vi "Main.vi"() -> ()   [LabVIEW 2014, in "GenNet-Client.lvlib"]
doc: "The GenNet-Client module is instantiated from a DQMH Generic Networking Module\nin order to forward messages via TCP/IP.\n\nThe GenNet-Client module forwards all requests to another DQMH Generic Networking \nModule running in another application and/or another PC accessible via TCP/IP.\n\n<b>Note:</b> This VI was modified by the <b>Validate DQMH Module</b> tool to upgrade it to the DQMH 5.0 approach to destroying cloneable module event references.\n\n<b>Note:</b> This VI was modified by the <b>Validate DQMH Module</b> tool to have the module name be passed as the Additional Information parameter with an Error Reported broadcast.\n\n<b>Note:</b> This VI was modified by the <b>Validate DQMH Module</b> tool to call the Release Message Queue VI in the top-level Error case.\n\n<b>Note:</b> This VI was modified by the <b>Validate DQMH Module</b> tool to call the Release Message Queue VI in the top-level Error case."
uses:
  GenNet-Client.lvlib
  <vilib>/Delacor/Delacor QMH/Libraries/Cloneable Module Admin_class/Delacor_lib_QMH_Cloneable Module Admin.lvclass
  DQMH-GenNet Message Queue.lvclass
  hse-dqmh/Controls/System Message Argument--cluster.ctl
  hse-dqmh/Controls/System Message Source.ctl
  Module Data--cluster.ctl
  Stop Argument--cluster.ctl
  <vilib>/Delacor/Delacor QMH/Libraries/Message Queue_class/Delacor_lib_QMH_Message Queue.lvclass/Delacor_lib_QMH_Message Queue.ctl
  <vilib>/Delacor/Delacor QMH/Libraries/Cloneable Module Admin_class/Delacor_lib_QMH_Cloneable Module Admin.lvclass/Delacor_lib_QMH_Cloneable Module Admin.ctl
  <vilib>/Delacor/Delacor QMH/Libraries/Module Admin_class/Delacor_lib_QMH_Module Admin.lvclass/Delacor_lib_QMH_Module Admin.ctl
  Connect Argument--cluster.ctl
  Connect (Reply Payload)--cluster.ctl
  Send via Network Argument--cluster.ctl
  Listen for Network Broadcasts Argument--cluster.ctl
  <vilib>/Utility/miscctls.llb/LVPointTypeDef.ctl
  <vilib>/Delacor/Delacor QMH/Libraries/Message Queue_class/Delacor_lib_QMH_Enqueue Message (Single).vi
  <vilib>/Delacor/Delacor QMH/Libraries/Cloneable Module Admin_class/Delacor_lib_QMH_Get Module ID.vi
  <vilib>/Delacor/Delacor QMH/Libraries/Module Admin_class/Delacor_lib_QMH_Get External Launch.vi
  <vilib>/Utility/tcp.llb/UDP Multicast Read-Only Open.vi
  <vilib>/Utility/error.llb/Error Cluster From Error Code.vi
  <vilib>/ErrorRing/Error Ring.xnode
  <vilib>/Delacor/Delacor QMH/Libraries/Message Queue_class/Delacor_lib_QMH_Message Queue.lvclass
  hse-gennet.lvlib
  hse-dqmh/hse-dqmh.lvlib
panel:
  in  "Call Chain":string[](array[string])
  in  "Caller SystemMsg":refnum<user-event>
  in  "Caller MsgQ":refnum<class "DQMH-GenNet Message Queue.lvclass">
  out "error out":errorcluster
  in  "Module Admin":refnum<class "Delacor_lib_QMH_Cloneable Module Admin.lvclass">
  # "The GenNet-Client module is instantiated from a DQMH Generic Networking Module\nin order to forward messages via TCP/IP.\n\nThe GenNet-Client module forwards all requests to another DQMH Generic Networking \nModule running in another application and/or another PC accessible via TCP/IP."
  # "hse-lib.lvlib:System Message Argument--cluster.ctlCaveat:\nThe Caller's message queue, which should be private to the caller only, is avail-\nable to the GenNet-Server module so that it can write messages directly. As the GenNet-Server\nmodule cannot be accessed from other code, and as messages that arrive via\nnetwork are to be considered local, this excemption to the rule is tolerable."
  # "Please get in touch with us at office@hampel-soft.com or visit our website www.hampel-soft.com"
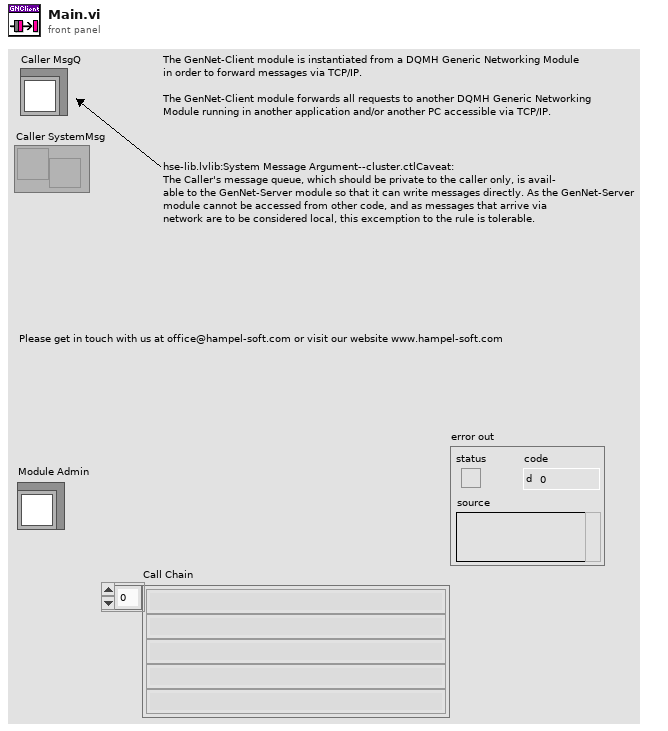
[diagram p1: front panel]
types:
  T1 = typedef "GenNet-Client.lvlib/Request Events--cluster.ctl" = cluster{"Stop Module":refnum<user-event>, "Show Panel":refnum<user-event>, "Hide Panel":refnum<user-event>, "Show Diagram":refnum<user-event>, "Get Module Execution Status":refnum<user-event>, "Send via Network":refnum<user-event>, "Connect":refnum<user-event>, "Listen for Network Broadcasts":refnum<user-event>}
  T2 = typedef "GenNet-Client.lvlib/Module Data--cluster.ctl" = cluster{"Status":string, "IP":string, "Port":u16, "Timeout":i32, "ConnID":refnum<k5>, "UDP ConnID":refnum<k16>, "TCP error":errorcluster}
  T3 = enum32{"invalid lock state", "Not Locked", "Locked (No Password)", "Password-protected"}
  T4 = typedef "GenNet-Client.lvlib/Stop Argument--cluster.ctl" = cluster{"Origin":string, "Module ID":i32, "Exit via Stop Module Req?":bool, "Wait for Module to stop?":bool}
  T5 = typedef "GenNet-Client.lvlib/Connect Argument--cluster.ctl" = cluster{"Module ID":i32, "Wait Notifier":refnum<notifier>}
  T6 = typedef "GenNet-Client.lvlib/Send via Network Argument--cluster.ctl" = cluster{"Module ID":i32, "Message Data":variant}
  T7 = typedef "hse-dqmh.lvlib/System Message Argument--cluster.ctl" = cluster{"Identifier":string, "Payload":variant, "Source Type":T8, "Source Name":string}
  T8 = typedef "hse-dqmh.lvlib/System Message Source.ctl" = enum16{"module", "application", "network"}
  T9 = typedef "GenNet-Client.lvlib/Listen for Network Broadcasts Argument--cluster.ctl" = cluster{"Module ID":i32, "Multicast Address":string, "Port":u16, "Local IP Address":string, "Max Rx Byte Size":i32}
  T10 = typedef "LVPointTypeDef.ctl" = cluster{"Horizontal":i16, "Vertical":i16}
  T11 = enum32{"Invalid", "Standard", "Closed", "Hidden", "Minimized", "Maximized"}
  T12 = typedef "GenNet-Client.lvlib/Connect (Reply Payload)--cluster.ctl" = cluster{"error":errorcluster}
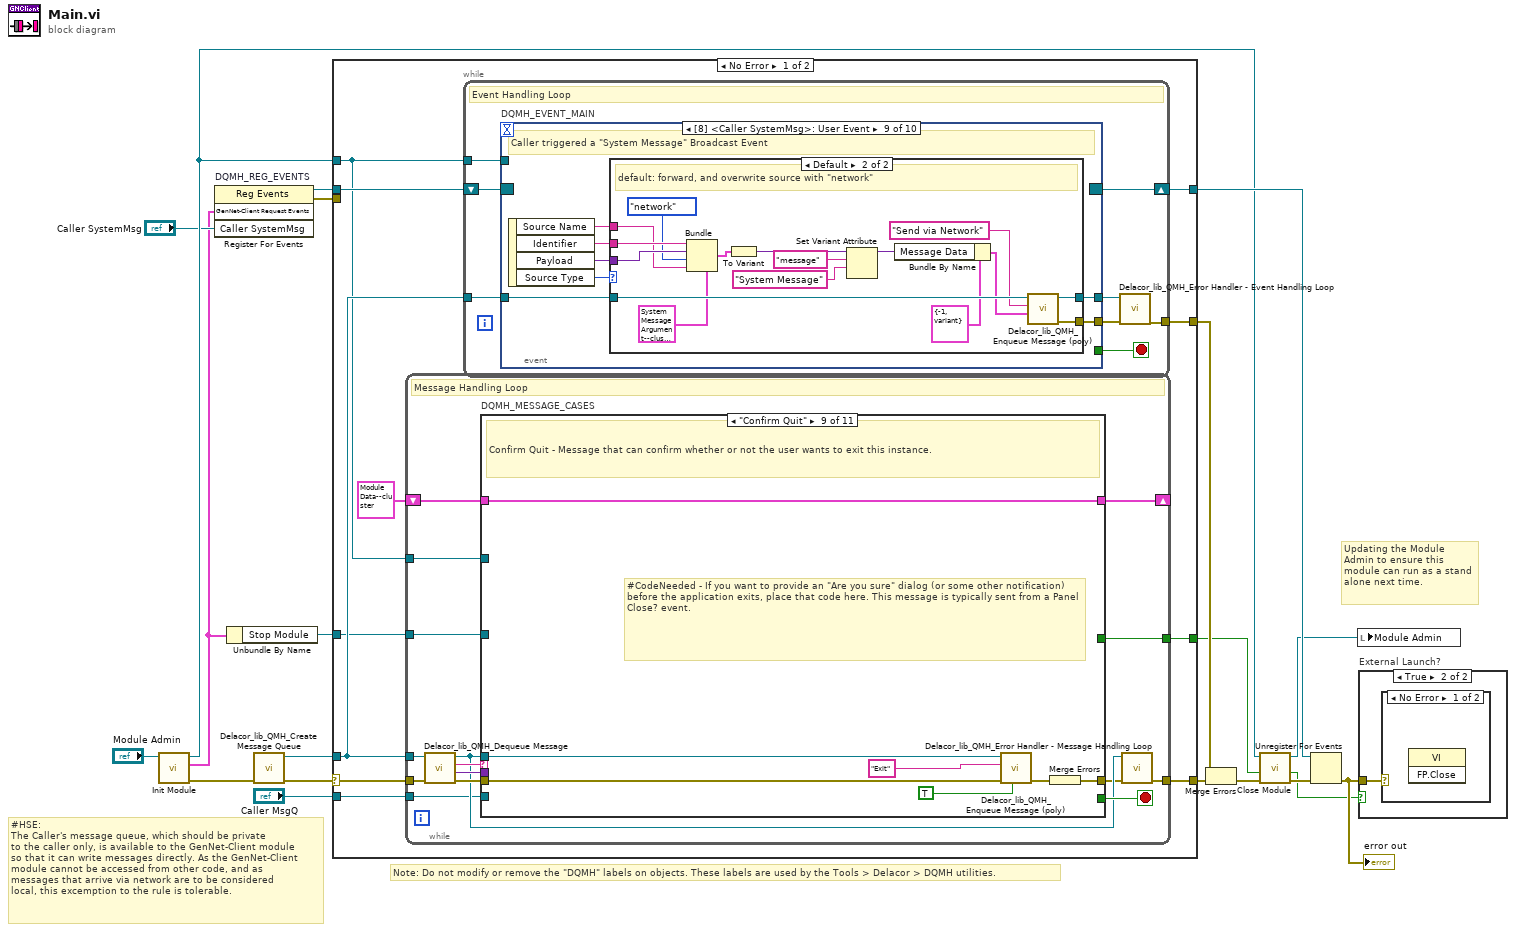
[diagram p0: block diagram]
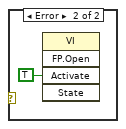
[diagram p3: hidden frame]
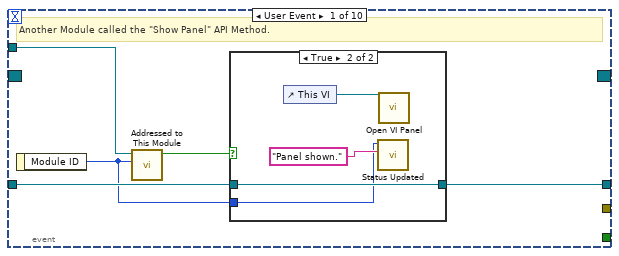
[diagram p4: hidden frame]
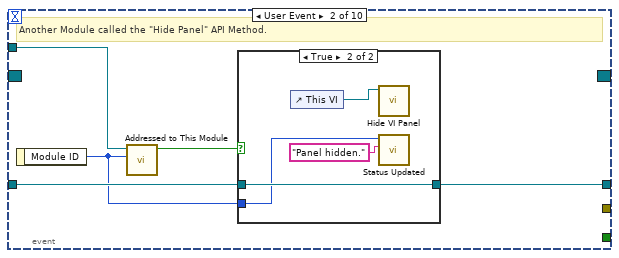
[diagram p6: hidden frame]
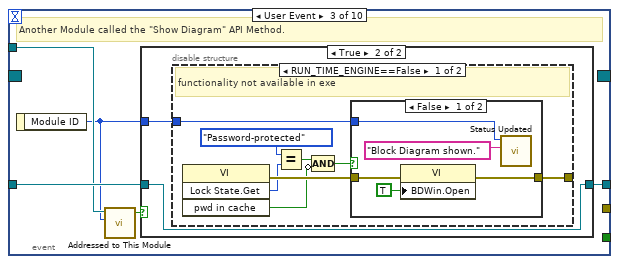
[diagram p8: hidden frame]
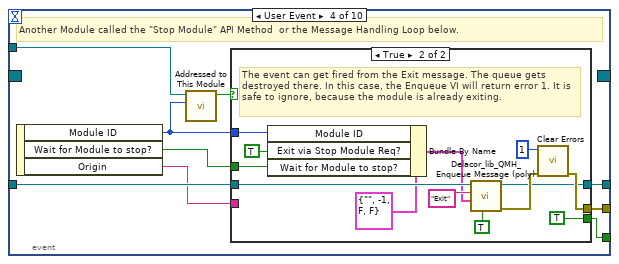
[diagram p12: hidden frame]
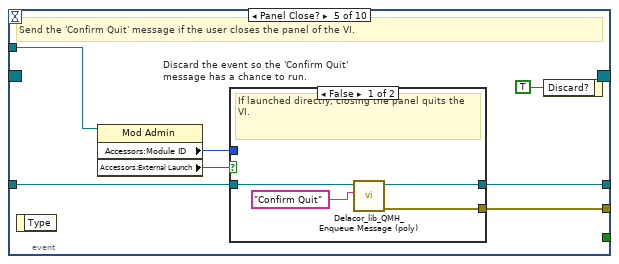
[diagram p14: hidden frame]
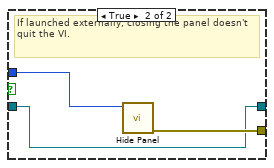
[diagram p15: hidden frame]
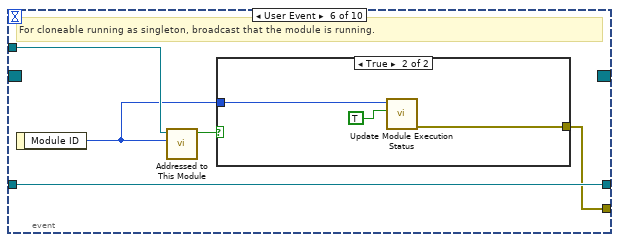
[diagram p16: hidden frame]
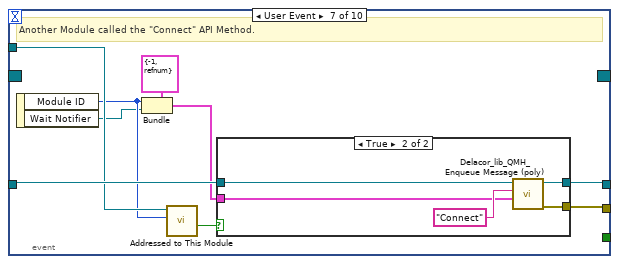
[diagram p18: hidden frame]
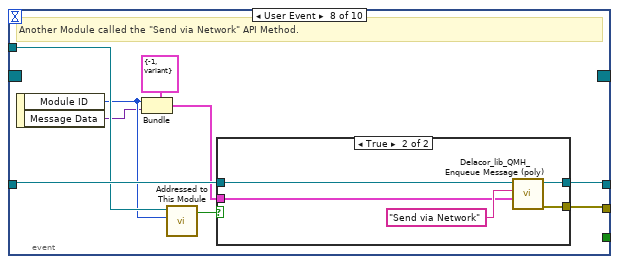
[diagram p20: hidden frame]
diagram:
  # "#HSE: \nThe Caller's message queue, which should be private \nto the caller only, is available to the GenNet-Client module \nso that it can write messages directly. As the GenNet-Client\nmodule cannot be accessed from other code, and as \nmessages that arrive via network are to be considered \nlocal, this excemption to the rule is tolerable."
  # "Note: Do not modify or remove the \"DQMH\" labels on objects. These labels are used by the Tools > Delacor > DQMH utilities."
  # "Updating the Module Admin to ensure this module can run as a stand alone next time."
  n1 = call "Init Module.vi"("Cloneable Module Admin in"="Module Admin") -> ("error out"=w17:errorcluster, "GenNet-Client Request Events"=w2:T1, "Cloneable Module Admin out"=w11:refnum<class "Delacor_lib_QMH_Cloneable Module Admin.lvclass">)  [unwired: 8 in]
  n2 = register-events "DQMH_REG_EVENTS"(w2, "Caller SystemMsg") -> (reference out=w15:refnum<event-registration>, error out=w4:errorcluster)  [unwired: 2 in]
  n3 = Unbundle By Name(w2) -> ("Stop Module"=w1:refnum<user-event>)
  n4 = call <vilib>:"Delacor_lib_QMH_Create Message Queue.vi"("error in (no error)"=w17) -> ("error out"=w6:errorcluster, "Message Queue"=w14:refnum<class "Delacor_lib_QMH_Message Queue.lvclass">)  [unwired: 9 in]
  n5 = case shown="No Error" w6 {
    selector: w6 -> [w25 w377]
    tunnel: [w31 w377] -> w18
    tunnel: [w30 w378] -> w16
    tunnel: w15 -> [w28 w378]
    tunnel: w14 -> [w27 w370]
    tunnel: [w26 _] -> w19
    tunnel: w11 -> [w24 w373]
    tunnel: [w23 _] -> w9
    tunnel: "Caller MsgQ" -> [w22 w369]
    tunnel: w4 -> [_ _]
    tunnel: w1 -> [w21 _]
    frame No Error {
      n6 = while {
        tunnel: w27 -> [w207]
        shift-right: [w213] -> _
        shift-left: T2 {"Status"="", "IP"="", "Port"=0, "Timeout"=0, "ConnID"=refnum, "UDP ConnID"=refnum, "TCP error"={"status"=FALSE, "code"=0, "source"=""}} ("Data Cluster") -> [w200]
        tunnel: w25 -> [w211]
        tunnel: [w205] -> w31
        tunnel: w24 -> [w204]
        tunnel: [w203] -> w23
        tunnel: w22 -> [w202]
        tunnel: w21 -> [w199]
        stop <- w212 stop-if-true
        # "Message Handling Loop"
        n7 = call-dynamic "Delacor_lib_QMH_Dequeue Message.vi"("error in (no error)"=w211, "Message Queue in"=w207) -> ("error out"=w210:errorcluster, "Message Data"=w208:variant, "Message"=w209:string, "Message Queue out"=w206:refnum<class "Delacor_lib_QMH_Message Queue.lvclass">)  [unwired: 6 in]
        n8 = case "DQMH_MESSAGE_CASES" shown="\"Confirm Quit\"" w209 {
          selector: w209 -> [_ _ _ _ _ _ _ _ _ _ w358]
          tunnel: w206 -> [_ _ _ _ _ _ _ w303 w322 w352 _]
          tunnel: w210 -> [w228 w243 w249 w273 w294 w297 w300 w312 w321 w354 _]
          tunnel: [w214 w241 w251 w266 w276 w295 w298 w302 w320 w338 w359] -> w201
          tunnel: w200 -> [w221 w242 w246 w264 w289 w296 w299 w311 w325 w339 w360]
          tunnel: [w221 w242 w247 w270 w288 w296 w299 w311 w325 w341 w360] -> w213
          tunnel: [_ _ _ _ _ _ _ _ _ w351 _] -> w212
          tunnel: w208 -> [_ _ w255 w272 w293 _ _ w310 _ w346 _]
          tunnel: w204 -> [w224 _ w258 _ w282 _ _ w307 _ w337 w356]
          tunnel: [_ _ _ _ _ _ _ _ _ w344 _] -> w203
          tunnel: w202 -> [_ _ w244 w267 w283 _ _ _ _ w326 _]
          tunnel: w199 -> [_ _ _ _ w284 _ _ _ _ _ _]
          frame "Initialize" {
            # "Initialize - Any operation that needs to be done before the module can receive messages. Synchronize Caller Events.vi will inform Start Module.vi that the module has launched and is ready to receive messages. Module Did Init.vi will broadcast that the module initialized."
            n9 = call "Synchronize Caller Events.vi"("error in (no error)"=w228, "Module Admin"=w224) -> ("error out"=w226:errorcluster, "Module Admin out"=w223:refnum<class "Delacor_lib_QMH_Cloneable Module Admin.lvclass">)  [unwired: 8 in]
            n10 = property class="Mod Admin"(reference=w223) -> ("Accessors:Module ID"=w222:i32, "Accessors:External Launch"=w225:bool)  [unwired: 1 in, 2 out]
            n11 = call "Module Name--constant.vi"("Module ID"=w222) -> ("Module Name"=w229:string)  [unwired: 10 in]
            n12 = call "Module Did Init.vi"("error in (no error)"=w226, "Initialized?"=TRUE, "Origin"=w229, "Module ID"=w222) -> ("error out"=w214:errorcluster)  [unwired: 7 in]
            n13 = disable-structure shown="TARGET_TYPE==Windows||EMBEDDED_UI==True" {
              disable-tunnel: w222 -> [w232 _]
              disable-tunnel: w225 -> [w230 _]
              frame condition #0 (active) {
                n14 = call "Module Name--constant.vi"("Module ID"=w232) -> ("Module Name"=w236:string)  [unwired: 10 in]
                n15 = property class="VI"("Front Panel.Title"=w236) -> (reference out=w239:refnum<vi>, error out=w240:errorcluster)  [unwired: 2 in]
                n16 = Select(t=T11."Hidden" ("State"), s=w230, f=T11."Standard" ("State")) -> (s? t:f=w233:T11)
                n17 = invoke class="VI" method="FP.Open"(reference=w239, error in=w240, "State"=w233) -> (reference out=w238:refnum<vi>, error out=w237:errorcluster)  [unwired: 2 in, 3 out]
                n18 = invoke class="VI" method="FP.Center"(reference=w238, error in=w237) -> ()  [unwired: 1 in, 3 out]
                n19 = property on="Pane" class="Pane"("Origin"=T10 {"Horizontal"=0, "Vertical"=0}) -> ()  [unwired: 2 in, 2 out]
              }
              frame condition #1 {
              }
            }
            n20 = Reverse 1D Array(array="Call Chain") -> (reversed array=w217:string[])
            n21 = Index Array(array=w217) -> (element=w218:string)  [unwired: 1 in]
            n22 = Match Pattern(string=w218, regular expression=".lvlib") -> (before substring=w215:string)  [unwired: 1 in, 3 out]
            n23 = Format Into String(format string="%s initialised from %s", w229, w215) -> ()  [unwired: 2 in, 2 out]
          }
          frame "--- Module Specific ---" {
            # "Separator -- The following cases handle messages specific to this Module."
            n24 = Merge Errors(w243) -> (w241:errorcluster)
          }
          frame "Connect" {
            # "Open the TCP/IP connection to the GenNet Server"
            n25 = Variant To Data(error in=w249, type=T5 {"Module ID"=-1, "Wait Notifier"=refnum} ("Connect Argument"), Variant=w255) -> (data=w256:T5, error out=w248:errorcluster)
            n26 = property class="Mod Admin"(reference=w258) -> ("Accessors:Module ID"=w245:i32)  [unwired: 1 in, 2 out]
            n27 = Unbundle By Name(w256) -> ("Wait Notifier"=w259:refnum<notifier>)
            n28 = call "Establish Connection.vi"("Caller's Queue In"=w244, "Module ID"=w245, "Data Cluster"=w246) -> ("error out"=w252:errorcluster, "Data Cluster out"=w247:T2)  [unwired: 7 in]
            n29 = Bundle By Name(cluster=T12 {"error"={"status"=FALSE, "code"=0, "source"=""}} ("Connect (Reply Payload)"), "error"=w252) -> (w254:T12)
            n30 = Send Notification(notification=w254, notifier=w259) -> (error out=w250:errorcluster)  [unwired: 1 in, 1 out]
            n31 = Merge Errors(w248, w250) -> (w251:errorcluster)
          }
          frame "Send via Network" {
            # "Forwards the message of a DQMH module via Network"
            n32 = Variant To Data(error in=w273, type=T6 {"Module ID"=-1, "Message Data"=variant} ("Send via Network Argument"), Variant=w272) -> (data=w260:T6, error out=w268:errorcluster)
            n33 = Unbundle By Name(w264) -> ("IP"=w261:string, "Port"=w262:u16, "Timeout"=w263:i32)
            n34 = call "GetNet-Client Check Network Parameters.vi"("error in (no error)"=w268, "Timeout"=w263, "Port"=w262, "IP"=w261) -> ("error out"=w269:errorcluster)  [unwired: 7 in]
            n35 = call "GetNet-Client Send Message.vi"("error in"=w269, "Send via Network Argument"=w260, "Data Cluster in"=w264) -> ("error out"=w265:errorcluster, "Data Cluster out"=w270:T2)  [unwired: 7 in]
            n36 = call "GenNet-Client Report Error.vi"("Caller MsgQ"=w267, "error in"=w265) -> ("error out"=w266:errorcluster)  [unwired: 9 in]
          }
          frame "Listen for Network Broadcasts" {
            # "Opens a port to listen for broadcasts sent by other modules via UDP"
            n37 = Variant To Data(error in=w294, type=T9 {"Module ID"=-1, "Multicast Address"="", "Port"=0, "Local IP Address"="", "Max Rx Byte Size"=10000} ("Listen for Network Broadcasts Argument"), Variant=w293) -> (data=w291:T9, error out=w277:errorcluster)
            n38 = property class="Mod Admin"(reference=w282) -> ("Accessors:Module ID"=w281:i32)  [unwired: 1 in, 2 out]
            n39 = Unbundle By Name(w291) -> ("Max Rx Byte Size"=w274:i32, "Local IP Address"=w275:string, "Port"=w278:u16, "Multicast Address"=w279:string)
            n40 = String To IP(1:w275) -> (0:w290:u32)
            n41 = String To IP(1:w279) -> (0:w287:u32)
            n42 = call-poly <vilib>:"UDP Multicast Open.vi"("net address"=w290, "error in (no error)"=w277, "multicast addr"=w287, "port"=w278) -> ("error out"=w285:errorcluster, "connection ID"=w286:refnum<k16>)  [unwired: 5 in, 1 out]
            n43 = call "NET-RX Spawn UDP Service.vi"("Max Rx Byte Size"=w274, "Module ID"=w281, "error in"=w285, "Caller MsgQ"=w283, "Stop Module"=w284, "UDP Connection ID"=w286) -> ("error out"=w276:errorcluster)  [unwired: 5 in]
            n44 = Bundle By Name(cluster=w289, "UDP ConnID"=w286) -> (w288:T2)
            n45 = Format Into String(format string="UDP Receiver created on Port %d and IP %s, Max Rx Byte Size = %d", w278, w279, w274) -> ()  [unwired: 2 in, 2 out]
          }
          frame "---Copy This Frame---" {
            # "Duplicate this frame when creating new messages.  Change this comment in the duplicated frame to describe this message."
            n46 = Merge Errors(w297) -> (w295:errorcluster)
          }
          frame "--- Exit and Error Handling---" {
            # "Separator - the following cases handle errors and exit messages."
            n47 = Merge Errors(w300) -> (w298:errorcluster)
          }
          frame "Error" {
            # "Error - Check the error message data and respond accordingly. This message is sent by the \"Error Handler\" VIs at the end of each loop in this application."
            n48 = property class="Mod Admin"(reference=w307) -> ("Accessors:External Launch"=w304:bool, "Accessors:Module ID"=w306:i32)  [unwired: 1 in, 2 out]
            n49 = Variant To Data(error in=w312, type=errorcluster {"status"=FALSE, "code"=0, "source"=""} ("error constant"), Variant=w310) -> (data=w313:errorcluster, error out=w308:errorcluster)
            n50 = call "Module Name--constant.vi"("Module ID"=w306) -> ("Module Name"=w301:string)  [unwired: 10 in]
            n51 = call "Error Reported.vi"("Additional Information"=w301, "Error"=w313, "Module ID"=w306) -> ()  [unwired: 8 in, 1 out]
            n52 = case shown="False" w304 {
              tunnel: [w318 _] -> w305
              tunnel: w303 -> [w317 _]
              tunnel: w313 -> [w314 _]
              frame False {
                # "If the module is running standalone, then pop up an error dialog and call the \"Exit\" message."
                n53 = call <vilib>:"Simple Error Handler.vi"("error in (no error)"=w314) -> ()  [unwired: 4 in, 5 out]
                n54 = call-poly <vilib>:"Delacor_lib_QMH_Enqueue Message (poly).vi"("Priority Message? (F)"=TRUE, "Message"="Exit", "Message Queue in"=w317) -> ("error out"=w318:errorcluster)  [unwired: 7 in, 1 out]
              }
              frame True {
                # "If the module was launched externally, calling the Error Reported broadcast VI is the only action performed by the \"Error\" message. The module's caller can then process the error appropriately."
              }
            }
            n55 = Merge Errors(w308, w305) -> (w302:errorcluster)
            n56 = local write "error out"(w302) -> ()
          }
          frame "Confirm Quit" {
            # "#CodeNeeded - If you want to provide an \"Are you sure\" dialog (or some other notification) before the application exits, place that code here. This message is typically sent from a Panel Close? event."
            # "Confirm Quit - Message that can confirm whether or not the user wants to exit this instance."
            n57 = call-poly <vilib>:"Delacor_lib_QMH_Enqueue Message (poly).vi"("Priority Message? (F)"=TRUE, "error in (no error)"=w321, "Message"="Exit", "Message Queue in"=w322) -> ("error out"=w324:errorcluster)  [unwired: 6 in, 1 out]
            n58 = Merge Errors(w324) -> (w320:errorcluster)
          }
          frame "Exit" {
            w348 = 91  # 91: not all Exit messages will have an argument
            w351 = TRUE  # Stop the VI
            # "Release the message queue reference"
            # "Exit - Exit the application."
            n59 = Unbundle By Name(w339) -> ("ConnID"=w342:refnum<k5>, "UDP ConnID"=w332:refnum<k16>)
            n60 = Variant To Data(error in=w354, type=T4 {"Origin"="", "Module ID"=-1, "Exit via Stop Module Req?"=FALSE, "Wait for Module to stop?"=FALSE} ("Stop Argument"), Variant=w346) -> (data=w335:T4, error out=w347:errorcluster)
            n61 = call "GenNet Close Connection.vi"("TCP Network Connection in"=w342) -> ("TCP Network Connection out"=w340:refnum<k5>)  [unwired: 9 in, 1 out]
            n62 = call "GenNet Close UDP Connection.vi"("UDP Network Connection in"=w332) -> ("UDP Network Connection out"=w333:refnum<k16>)  [unwired: 9 in, 1 out]
            n63 = Bundle By Name(cluster=w339, "ConnID"=w340, "UDP ConnID"=w333) -> (w341:T2)
            n64 = call <vilib>:"Clear Errors.vi"("error in (no error)"=w347, "specific error code to clear (0: all)"=w348) -> ("error out"=w353:errorcluster)  [unwired: 4 in, 1 out]
            n65 = control-ref of="This VI"() -> (w343:refnum<vi>)
            n66 = call "Handle Exit.vi"("Stop Argument"=w335, "Module Admin in"=w337, "VI reference"=w343) -> ("error out"=w349:errorcluster, "Wait for Stop?"=w344:bool)  [unwired: 7 in]
            n67 = call-dynamic "Delacor_lib_QMH_Release Message Queue.vi"("error in (no error)"=w353, "Message Queue"=w352) -> ("error out"=w350:errorcluster)  [unwired: 9 in]
            n68 = Merge Errors(w349, w350) -> (w338:errorcluster)
            n69 = property class="Mod Admin"(reference=w337) -> ("Accessors:Module ID"=w336:i32)  [unwired: 1 in, 2 out]
            n70 = Unbundle By Name(w335) -> ("Origin"=w334:string)
            n71 = call "Module Name--constant.vi"("Module ID"=w336) -> ("Module Name"=w327:string)  [unwired: 10 in]
            n72 = call "GenNet Format System Message for MsgQ.vi"("Source Name"=w327, "Identifer"="Client disconnected and exited." ("Message")) -> ("System Message Argument"=w330:T7, "System Message constant"=w331:string)  [unwired: 8 in]
            n73 = Format Into String(format string="%s stopped (%s).", w327, w334) -> ()  [unwired: 2 in, 2 out]
            n74 = call-poly <vilib>:"Delacor_lib_QMH_Enqueue Message (poly).vi"("Message Data"=w330, "Message"=w331, "Message Queue in"=w326) -> ()  [unwired: 7 in, 2 out]
          }
          frame Default {
            # "'Default' case only runs if there is a message that isn't defined in any of the other cases.  Output a programming error."
            n75 = property class="Mod Admin"(reference=w356) -> ("Accessors:Module ID"=w355:i32)  [unwired: 1 in, 2 out]
            n76 = call "Module Name--constant.vi"("Module ID"=w355) -> ("Module Name"=w357:string)  [unwired: 10 in]
            n77 = xnode "Error Ring"("parameter 0"=w358, "parameter 1"=w357) -> ("error out"=w359:errorcluster)
          }
        }
        n78 = call-dynamic "Delacor_lib_QMH_Error Handler - Message Handling Loop.vi"("error in (no error)"=w201, "Message Queue in"=w206) -> ("dup error in"=w205:errorcluster)  [unwired: 8 in, 1 out]
      }
      n79 = while {
        tunnel: w27 -> [w39]
        shift-right: [w37] -> w30
        shift-left: w28 -> [w38]
        tunnel: [w33] -> w26
        tunnel: w24 -> [w32]
        stop <- w35 stop-if-true
        # "Event Handling Loop"
        n80 = event "DQMH_EVENT_MAIN" shown="[8] <Caller SystemMsg>: User Event" {
          selector: w38 -> [_ _ _ _ _ _ _ _ _ _]
          dyn-events: [_ _ _ _ _ _ _ _ _ _] -> w37
          timeout: _ -> [_ _ _ _ _ _ _ _ _ _]
          tunnel: [_ _ _ w85 _ _ _ _ _ _] -> w35
          tunnel: w39 -> [w44 w54 w64 w88 w110 w121 w135 w150 w163 w192]
          tunnel: [_ _ _ w90 w109 w120 w127 w142 w161 w183] -> w36
          tunnel: [w43 w53 w63 w89 w108 w121 w134 w149 w162 w191] -> w34
          tunnel: w32 -> [w41 w51 w61 w87 w107 w122 w132 w147 _ w189]
          event User Event {
            # "Another Module called the \"Show Panel\" API Method."
            n81 = event-data() -> ("Module ID"=w40:i32)  [unwired: 1 in]
            n82 = call "Addressed to This Module.vi"("Module ID from Argument"=w40, "Module Admin"=w41) -> ("Addressed to this instance?"=w42:bool)  [unwired: 8 in, 1 out]
            n83 = case shown="True" w42 {
              tunnel: w44 -> [w45 w49]
              tunnel: [w45 w49] -> w43
              tunnel: w40 -> [_ w46]
              frame False {
              }
              frame True {
                n84 = control-ref of="This VI"() -> (w47:refnum<vi>)
                n85 = call "Status Updated.vi"("Status"="Panel shown." ("format string"), "Module ID"=w46) -> ()  [unwired: 9 in, 1 out]
                n86 = call "Open VI Panel.vi"("VI"=w47) -> ()  [unwired: 10 in, 1 out]
              }
            }
          }
          event User Event {
            # "Another Module called the \"Hide Panel\" API Method."
            n87 = event-data() -> ("Module ID"=w50:i32)  [unwired: 1 in]
            n88 = call "Addressed to This Module.vi"("Module ID from Argument"=w50, "Module Admin"=w51) -> ("Addressed to this instance?"=w52:bool)  [unwired: 8 in, 1 out]
            n89 = case shown="True" w52 {
              tunnel: w54 -> [w55 w59]
              tunnel: [w55 w59] -> w53
              tunnel: w50 -> [_ w57]
              frame False {
              }
              frame True {
                n90 = control-ref of="This VI"() -> (w56:refnum<vi>)
                n91 = call "Hide VI Panel.vi"("VI"=w56) -> ()  [unwired: 10 in, 1 out]
                n92 = call "Status Updated.vi"("Status"="Panel hidden." ("format string"), "Module ID"=w57) -> ()  [unwired: 9 in, 1 out]
              }
            }
          }
          event User Event {
            # "Another Module called the \"Show Diagram\" API Method."
            n93 = event-data() -> ("Module ID"=w60:i32)  [unwired: 1 in]
            n94 = call "Addressed to This Module.vi"("Module ID from Argument"=w60, "Module Admin"=w61) -> ("Addressed to this instance?"=w62:bool)  [unwired: 8 in, 1 out]
            n95 = case shown="True" w62 {
              tunnel: w64 -> [w65 w66]
              tunnel: [w65 w66] -> w63
              tunnel: w60 -> [_ w67]
              frame False {
              }
              frame True {
                n96 = disable-structure shown="RUN_TIME_ENGINE==False" {
                  disable-tunnel: [w75 _] -> _
                  disable-tunnel: w67 -> [w68 _]
                  frame condition #0 (active) {
                    # "functionality not available in exe"
                    n97 = invoke class="VI" method="Lock State.Get"() -> (error out=w74:errorcluster, "Get Lock State"=w73:T3, "pwd in cache"=w70:bool)  [unwired: 4 in, 1 out]
                    n98 = Equal?(x=T3."Password-protected", y=w73) -> (x = y?=w71:bool)
                    n99 = Compound Arithmetic op=AND(w71, invert w70) -> (w69:bool)
                    n100 = case shown="False" w69 {
                      tunnel: [w79 w81] -> w75
                      tunnel: w74 -> [w78 w81]
                      tunnel: w68 -> [w76 _]
                      frame False {
                        n101 = property class="VI"(error in=w78, "BDWin.Open"=TRUE ("Block Diagram Window:Open")) -> (error out=w79:errorcluster)  [unwired: 1 in, 1 out]
                        n102 = call "Status Updated.vi"("Status"="Block Diagram shown." ("format string"), "Module ID"=w76) -> ()  [unwired: 9 in, 1 out]
                      }
                      frame True {
                        # "Password-protected VI, and the password is not in the cache. Do not show the diagram."
                      }
                    }
                  }
                  frame condition #1 {
                  }
                }
              }
            }
          }
          event User Event {
            # "Another Module called the \"Stop Module\" API Method  or the Message Handling Loop below."
            n103 = event-data() -> ("Module ID"=w83:i32, "Wait for Module to stop?"=w84:bool, "Origin"=w82:string)  [unwired: 1 in]
            n104 = call "Addressed to This Module.vi"("Module ID from Argument"=w83, "Module Admin"=w87) -> ("Addressed to this instance?"=w86:bool)  [unwired: 8 in, 1 out]
            n105 = case shown="True" w86 {
              tunnel: [_ w100] -> w90
              tunnel: [w91 w99] -> w89
              tunnel: w88 -> [w91 w98]
              tunnel: [_ TRUE] -> w85
              tunnel: w84 -> [_ w93]
              tunnel: w83 -> [_ w95]
              tunnel: w82 -> [_ _]
              frame False {
              }
              frame True {
                # "The event can get fired from the Exit message. The queue gets destroyed there. In this case, the Enqueue VI will return error 1. It is safe to ignore, because the module is already exiting."
                n106 = Bundle By Name(cluster=T4 {"Origin"="", "Module ID"=-1, "Exit via Stop Module Req?"=FALSE, "Wait for Module to stop?"=FALSE} ("Stop Argument"), "Module ID"=w95, "Exit via Stop Module Req?"=TRUE, "Wait for Module to stop?"=w93) -> (w92:T4)
                n107 = call-poly <vilib>:"Delacor_lib_QMH_Enqueue Message (poly).vi"("Priority Message? (F)"=TRUE, "Message Data"=w92, "Message"="Exit", "Message Queue in"=w98) -> ("error out"=w103:errorcluster, "Message Queue out"=w99:refnum<class "Delacor_lib_QMH_Message Queue.lvclass">)  [unwired: 6 in]
                n108 = call <vilib>:"Clear Errors.vi"("error in (no error)"=w103, "specific error code to clear (0: all)"=1) -> ("error out"=w100:errorcluster)  [unwired: 4 in, 1 out]
              }
            }
          }
          event Panel Close? {
            w111 = TRUE  # Discard the event so the 'Confirm Quit' message has a chance to run.
            # "Send the 'Confirm Quit' message if the user closes the panel of the VI."
            n109 = event-data() -> ()  [unwired: 1 in, 1 out]
            n110 = property class="Mod Admin"(reference=w107) -> ("Accessors:Module ID"=w105:i32, "Accessors:External Launch"=w106:bool)  [unwired: 1 in, 2 out]
            n111 = case shown="False" w106 {
              tunnel: w110 -> [w115 w116]
              tunnel: [w114 w118] -> w109
              tunnel: [w113 w116] -> w108
              tunnel: w105 -> [_ w117]
              frame False {
                # "If launched directly, closing the panel quits the VI."
                n112 = call-poly <vilib>:"Delacor_lib_QMH_Enqueue Message (poly).vi"("Message"="Confirm Quit", "Message Queue in"=w115) -> ("error out"=w114:errorcluster, "Message Queue out"=w113:refnum<class "Delacor_lib_QMH_Message Queue.lvclass">)  [unwired: 8 in]
              }
              frame True {
                # "If launched externally, closing the panel doesn't quit the VI."
                n113 = call "Hide Panel.vi"("Module ID"=w117) -> ("error out"=w118:errorcluster)  [unwired: 10 in]
              }
            }
            n114 = event-data("Discard?"=w111) -> ()  [unwired: 1 in, 1 out]
          }
          event User Event {
            # "For cloneable running as singleton, broadcast that the module is running."
            n115 = event-data() -> ("Module ID"=w119:i32)  [unwired: 1 in]
            n116 = call "Addressed to This Module.vi"("Module ID from Argument"=w119, "Module Admin"=w122) -> ("Addressed to this instance?"=w123:bool)  [unwired: 8 in, 1 out]
            n117 = case shown="True" w123 {
              tunnel: [_ w126] -> w120
              tunnel: w119 -> [_ w125]
              frame False {
              }
              frame True {
                n118 = call "Update Module Execution Status.vi"("Running?"=TRUE, "Module ID"=w125) -> ("error out"=w126:errorcluster)  [unwired: 9 in]
              }
            }
          }
          event User Event {
            # "Another Module called the \"Connect\" API Method."
            n119 = event-data() -> ("Module ID"=w129:i32, "Wait Notifier"=w128:refnum<notifier>)  [unwired: 1 in]
            n120 = Bundle(cluster=T5 {"Module ID"=-1, "Wait Notifier"=refnum} ("Connect Argument"), "Module ID"=w129, "Wait Notifier"=w128) -> (w130:T5)
            n121 = call "Addressed to This Module.vi"("Module ID from Argument"=w129, "Module Admin"=w132) -> ("Addressed to this instance?"=w133:bool)  [unwired: 8 in, 1 out]
            n122 = case shown="True" w133 {
              tunnel: w135 -> [w136 w141]
              tunnel: [w136 w140] -> w134
              tunnel: w130 -> [_ w138]
              tunnel: [_ w137] -> w127
              frame False {
              }
              frame True {
                n123 = call-poly <vilib>:"Delacor_lib_QMH_Enqueue Message (poly).vi"("Message Data"=w138, "Message"="Connect", "Message Queue in"=w141) -> ("error out"=w137:errorcluster, "Message Queue out"=w140:refnum<class "Delacor_lib_QMH_Message Queue.lvclass">)  [unwired: 7 in]
              }
            }
          }
          event User Event {
            # "Another Module called the \"Send via Network\" API Method."
            n124 = event-data() -> ("Module ID"=w144:i32, "Message Data"=w143:variant)  [unwired: 1 in]
            n125 = Bundle(cluster=T6 {"Module ID"=-1, "Message Data"=variant} ("Send via Network Argument"), "Module ID"=w144, "Message Data"=w143) -> (w145:T6)
            n126 = call "Addressed to This Module.vi"("Module ID from Argument"=w144, "Module Admin"=w147) -> ("Addressed to this instance?"=w148:bool)  [unwired: 8 in, 1 out]
            n127 = case shown="True" w148 {
              tunnel: w150 -> [w151 w156]
              tunnel: [w151 w155] -> w149
              tunnel: w145 -> [_ w153]
              tunnel: [_ w152] -> w142
              frame False {
              }
              frame True {
                n128 = call-poly <vilib>:"Delacor_lib_QMH_Enqueue Message (poly).vi"("Message Data"=w153, "Message"="Send via Network", "Message Queue in"=w156) -> ("error out"=w152:errorcluster, "Message Queue out"=w155:refnum<class "Delacor_lib_QMH_Message Queue.lvclass">)  [unwired: 7 in]
              }
            }
          }
          event User Event {
            # "Caller triggered a \"System Message\" Broadcast Event"
            n129 = event-data() -> ("Source Name"=w157:string, "Identifier"=w160:string, "Payload"=w159:variant, "Source Type"=w158:T8)  [unwired: 1 in]
            n130 = case shown="Default" w158 {
              tunnel: w163 -> [w164 w180]
              tunnel: [w164 w179] -> w162
              tunnel: [_ w178] -> w161
              tunnel: w160 -> [_ w174]
              tunnel: w159 -> [_ w173]
              tunnel: w157 -> [_ w165]
              frame "network" {
                # "do not forward messages from source \"network\""
              }
              frame Default {
                # "default: forward, and overwrite source with \"network\""
                n131 = Bundle(cluster=T7 {"Identifier"="", "Payload"=variant, "Source Type"=enum."module", "Source Name"=""} ("System Message Argument"), "Identifier"=w174, "Payload"=w173, "Source Type"=System_Message_Source."network" ("Source"), "Source Name"=w165) -> (w172:T7)
                n132 = To Variant(anything=w172) -> (Variant=w171:variant)
                n133 = Set Variant Attribute(Variant=w171, name="message", value="System Message" ("name")) -> (Variant out=w170:variant)  [unwired: 1 in, 2 out]
                n134 = Bundle By Name(cluster=T6 {"Module ID"=-1, "Message Data"=variant} ("Send via Network Argument"), "Message Data"=w170) -> (w175:T6)
                n135 = call-poly <vilib>:"Delacor_lib_QMH_Enqueue Message (poly).vi"("Message Data"=w175, "Message"="Send via Network", "Message Queue in"=w180) -> ("error out"=w178:errorcluster, "Message Queue out"=w179:refnum<class "Delacor_lib_QMH_Message Queue.lvclass">)  [unwired: 7 in]
              }
            }
          }
          event User Event {
            # "Another Module called the \"Listen for Network Broadcasts\" API Method."
            n136 = event-data() -> ("Module ID"=w186:i32, "Multicast Address"=w185:string, "Port"=w184:u16, "Local IP Address"=w182:string, "Max Rx Byte Size"=w181:i32)  [unwired: 1 in]
            n137 = Bundle(cluster=T9 {"Module ID"=-1, "Multicast Address"="", "Port"=0, "Local IP Address"="", "Max Rx Byte Size"=10000} ("Listen for Network Broadcasts Argument"), "Module ID"=w186, "Multicast Address"=w185, "Port"=w184, "Local IP Address"=w182, "Max Rx Byte Size"=w181) -> (w187:T9)
            n138 = call "Addressed to This Module.vi"("Module ID from Argument"=w186, "Module Admin"=w189) -> ("Addressed to this instance?"=w190:bool)  [unwired: 8 in, 1 out]
            n139 = case shown="True" w190 {
              tunnel: w192 -> [w193 w198]
              tunnel: [w193 w197] -> w191
              tunnel: w187 -> [_ w195]
              tunnel: [_ w194] -> w183
              frame False {
              }
              frame True {
                n140 = call-poly <vilib>:"Delacor_lib_QMH_Enqueue Message (poly).vi"("Message Data"=w195, "Message"="Listen for Network Broadcasts", "Message Queue in"=w198) -> ("error out"=w194:errorcluster, "Message Queue out"=w197:refnum<class "Delacor_lib_QMH_Message Queue.lvclass">)  [unwired: 7 in]
              }
            }
          }
        }
        n141 = call-dynamic "Delacor_lib_QMH_Error Handler - Event Handling Loop.vi"("error in (no error)"=w36, "Message Queue in"=w34) -> ("dup error in"=w33:errorcluster)  [unwired: 8 in, 1 out]
      }
    }
    frame Error {
      n142 = call "Synchronize Caller Events.vi"("Module Admin"=w373) -> ("Module Admin out"=w372:refnum<class "Delacor_lib_QMH_Cloneable Module Admin.lvclass">)  [unwired: 9 in, 1 out]
      n143 = property class="Mod Admin"(reference=w372) -> ("Accessors:Module ID"=w371:i32)  [unwired: 1 in, 2 out]
      n144 = call-dynamic "Delacor_lib_QMH_Release Message Queue.vi"("Message Queue"=w370) -> ()  [unwired: 10 in, 1 out]
      n145 = call-dynamic "Delacor_lib_QMH_Release Message Queue.vi"("Message Queue"=w369) -> ()  [unwired: 10 in, 1 out]
      n146 = call "Module Name--constant.vi"("Module ID"=w371) -> ("Module Name"=w376:string)  [unwired: 10 in]
      n147 = Format Into String(format string="An error occurred during initialization. %s is no longer running.", w376) -> (resulting string=w374:string)  [unwired: 2 in, 1 out]
      n148 = call "Error Reported.vi"("Additional Information"=w374, "Error"=w377, "Module ID"=w371) -> ()  [unwired: 8 in, 1 out]
    }
  }
  n149 = Merge Errors(w19, w18) -> (w20:errorcluster)
  n150 = call "Close Module.vi"("error in (no error)"=w20, "Wait for stop?"=w9, "Module Admin in"=w11) -> ("error out"=w13:errorcluster, "External Launch"=w7:bool, "Module Admin out"=w10:refnum<class "Delacor_lib_QMH_Cloneable Module Admin.lvclass">)  [unwired: 6 in]
  n151 = Unregister For Events(event registration refnum=w16, error in=w13) -> (error out=w8:errorcluster)
  "error out" <- w8
  n152 = local write "Module Admin"(w10) -> ()
  n153 = case "External Launch?" shown="True" w7 {
    tunnel: w8 -> [_ w379]
    frame False {
    }
    frame True {
      n154 = case shown="No Error" w379 {
        frame No Error {
          n155 = invoke class="VI" method="FP.Close"() -> ()  [unwired: 3 in, 3 out]
        }
        frame Error {
          n156 = invoke class="VI" method="FP.Open"("Activate"=TRUE ("Activate?")) -> ()  [unwired: 4 in, 5 out]
        }
      }
    }
  }
